vi "接收数据防呆.vi"(11 "重复数据输入":string) -> (3 "数据输出":string)   [LabVIEW 2020]
panel:
  out "error out":errorcluster
  out "数值":i32
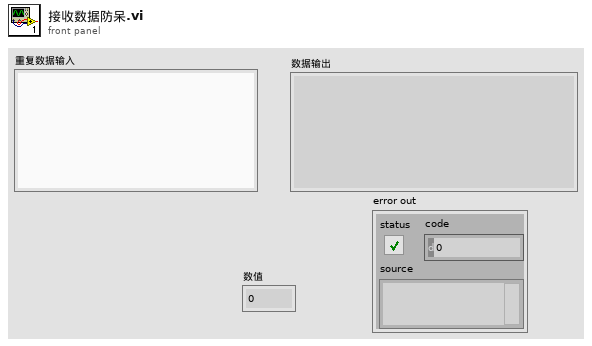
[diagram p1: front panel]
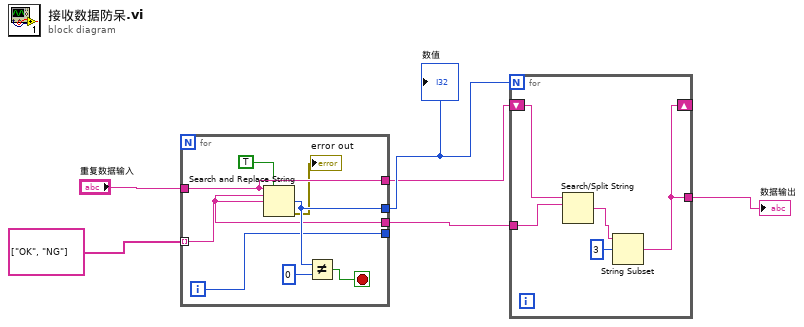
[diagram p0: block diagram]
diagram:
  n1 = for {
    tunnel: "重复数据输入" -> [w10]
    tunnel: string[] ["OK", "NG"] ("替换字符串(\"\")") -> [w9] mode=indexing
    tunnel: [w12] -> w4
    tunnel: [w11] -> _
    tunnel: [w10] -> w3
    tunnel: [w9] -> w5
    i -> [w11]
    stop <- w13 stop-if-true
    n2 = Search and Replace String(replace all?=TRUE ("替换全部？(F)"), input string=w10, search string=w9, replace string=w9) -> (number of replacements=w12:i32, error out=→"error out":errorcluster)  [unwired: 4 in, 2 out]
    n3 = Not Equal?(x=w12, y=0) -> (x != y?=w13:bool)
  }
  "数值" <- w4
  n4 = for {
    N: w4 -> [_]
    tunnel: w5 -> [w19]
    shift-right: [w15] -> _
    shift-left: w3 -> [w18]
    tunnel: [w15] -> w2
    n5 = Search/Split String(string=w18, search string/char (-)=w19) -> (match + rest of string=w16:string)  [unwired: 1 in, 2 out]
    n6 = String Subset(string=w16, offset (0)=3 ("偏移量(0)")) -> (substring=w15:string)  [unwired: 1 in]
  }
  "数据输出" <- w2
